vi "TLB Native Dynamic Events ver 0.07b.vi"() -> ()   [LabVIEW 2018]
uses:
  Labview Training Phase 2/Enum Controls/States for Action Engine.ctl
  Type def/TLB event states.ctl
  Type def/TLB MHL States.ctl
  <vilib>/Studica/Studica Toolkit/Background/I2C Channel.ctl
  <vilib>/Studica/Studica Toolkit/NavX/NavX.lvlib
  <vilib>/myRIO/Common/Instrument Driver Framework/myRIO v1.0/AI/typedefs/AI Channels Enum.ctl
  <vilib>/myRIO/Common/Instrument Driver Framework/myRIO v1.0/AI/typedefs/AI Channels List.ctl
  Type def/Type def.ctl
  Type def/Motor Control Cluster.ctl
  <vilib>/Studica/Studica Blackhawk/Blackhawk.lvlib
  <vilib>/userdefined/High Color/IMAQdx.ctl
  Underlying VI's/Webcam FGV Low level ver/State control.ctl
  <vilib>/Studica/Studica Toolkit/Background/Mxp Selection.ctl
  <vilib>/Studica/Studica Toolkit/Background/DIO Channel.ctl
  <vilib>/addons/control/pid/NI_PID_pid.lvlib
  <vilib>/addons/control/pid/pid.llb/PID (DBL).vi
  <vilib>/NI_Real-Time Target Support.lvlib
  <vilib>/ptbypt/NI_PtbyPt.lvlib
panel:
  out "Speed and distance cluster":T1
  out "Waveform Chart 2":dbl(graph)
  out "Load":errorcluster
  out "Waveform Chart":dbl(graph)
  in  "STOP":bool
  out "DIO 0":bool
  out "DIO 1":bool
  out "Limit Switch Array":bool[](array[boolean])
  out "error out":errorcluster
  out "L/R average":fxp<+,64,64>
  out "Right Ultrasonic":fxp<+,64,16>
  out "Left Ultrasonic":fxp<+,64,16>
  out "Object detection count":T2
  out "Camera error":errorcluster
  out "Right IR Sensor":dbl
  out "Left IR Sensor":dbl
  in  "Servo Angle":u8(slide) scale=0.0..180.0
  in  "On/Off":bool
  out "Blackhawk error":errorcluster
  out "element":T3
  out "Action Queue Items":i32
  out "State Logic Queue Items":i32
  out "Action Queues items":string[](array[string])=["Hardware reset", "Software reset", ""]
  out "State logic":T4=enum."Task 2"
  out "Action State":string
  in  "Tasks Selector":string(combo)="Drive straight"
  out "Yaw":dbl
  in  "NavX Zero Yaw":bool
  # "Camera Status Loop"
  # "TLB FRAMEWORK STATUS"
  # "Test Programme written by Calvin Loke    Dated: 28 Aug 2019\nTest Programme revised by Dr Alex See   Dated 30 Aug 2019\n\nProgramme version:   TLB Native Dynamic Events ver 0.04b.vi"
  # "Sequence of Actions"
  # "Continuous (Repeated)"
  # "Motor Control Loop"
  # "NAVX Control Loop"
  # "Sensor data"
  # "Blackhawk status"
  # "System Health Status Update"
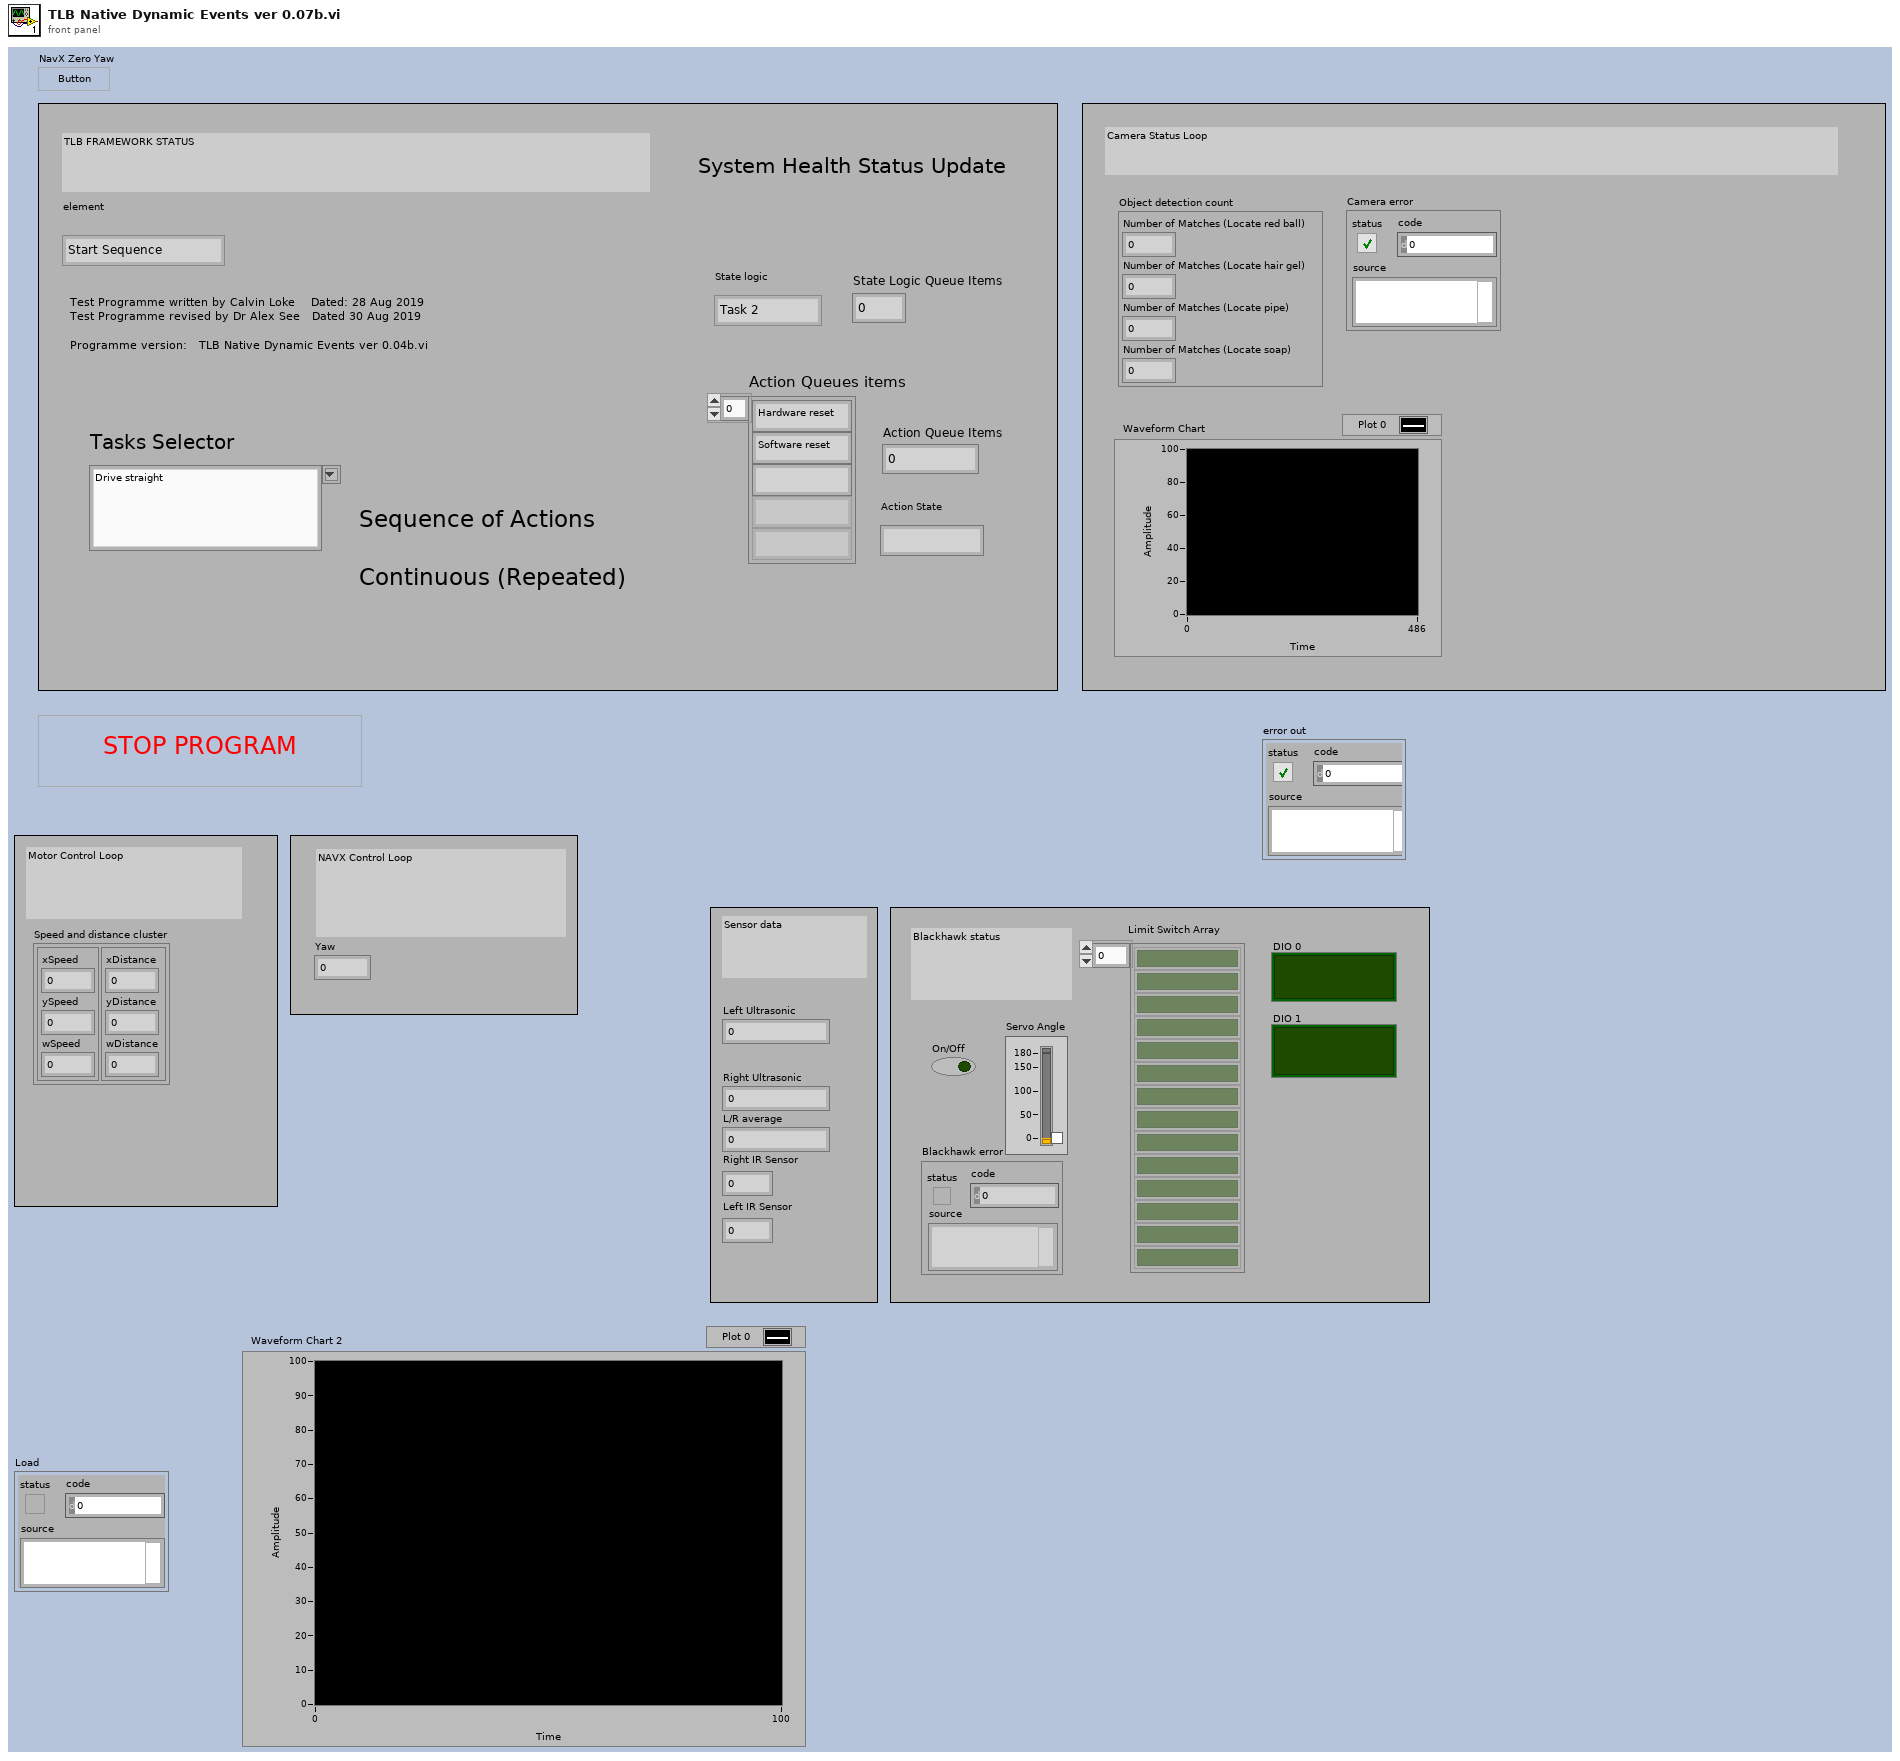
[diagram p1: front panel]
types:
  T1 = cluster{cluster{"xSpeed":dbl, "ySpeed":dbl, "wSpeed":dbl}, cluster{"xDistance":dbl, "yDistance":dbl, "wDistance":dbl}}
  T2 = cluster{"Number of Matches (Locate red ball)":i32, "Number of Matches (Locate hair gel)":i32, "Number of Matches (Locate pipe)":i32, "Number of Matches (Locate soap)":i32}
  T3 = typedef "TLB event states.ctl" = enum16{"Start Sequence", "Exit", "Start Task 1", "Start Task 2", "Start Task 3", "Start Task 4", "Camera vision", "Wall follow mode", "Idle", "Start Drive Straight"}
  T4 = typedef "TLB MHL States.ctl" = enum16{"None", "Startup", "Idle", "Processing", "Shutdown", "Reset", "Task 1", "Task 2", "Task 3", "Task 4", "Task 4a", "Task 4b", "Task 4c", "Task 4d", "Task 4e", "Task 4f", "Task 4g", "Task 4h", "Acquire image", "Wall follow mode", "Autodrive", "Autodrive a"}
  T5 = typedef "States for Action Engine.ctl" = enum16{"Initialize", "Write", "Read"}
  T6 = typedef "DIO Channel.ctl" = enum16{"Not Connected", "A/DIO1", "A/DIO2", "A/DIO3", "A/DIO4", "A/DIO5", "A/DIO6", "A/DIO7", "A/DIO13", "B/DIO1", "B/DIO2", "B/DIO3", "B/DIO4", "B/DIO5", "B/DIO6", "B/DIO7", "B/DIO13", "C/DIO0", "C/DIO1", "C/DIO2", "C/DIO3", "C/DIO4", "C/DIO5", "C/DIO6", "C/DIO7"}
  T7 = typedef "Motor Control Cluster.ctl" = cluster{"Vx":dbl, "Vy":dbl, "Vw":dbl}
  T8 = typedef "Type def.ctl" = cluster{"Front Ultrasonic Obstruct":bool, "Left Ultrasonic Obstruct":bool, "Right Ultrasonic Obstruct ":bool}
  T9 = typedef "I2C Channel.ctl" = enum16{"Not Connected", "A", "B"}
  T10 = typedef "TLB MHL States.ctl" = enum16{"None", "Startup", "Idle", "Processing", "Shutdown", "Reset", "Task 1", "Task 2", "Task 3", "Task 4", "Task 4a", "Task 4b", "Task 4c", "Task 4d", "Task 4e", "Task 4f", "Task 4g", "Task 4h", "Acquire image", "Wall follow mode", "Drive Straight"}
  T11 = cluster{"proportional gain (Kc)":dbl, "integral time (Ti, min)":dbl, "derivative time (Td, min)":dbl}
  T12 = typedef "State control.ctl" = enum16{"Initialise", "Start camera", "Continuous Acquisition ", "Stop camera", "Dispose all"}
  T13 = typedef "IMAQdx.ctl" = refnum<k21>
  T14 = typedef "Mxp Selection.ctl" = enum16{"MXP A", "MXP B"}
  T15 = cluster{"xTargetSpeed":dbl, "yTargetSpeed":dbl, "wTargetSpeed":dbl}
  T16 = typedef "IMAQ Image.ctl" = refnum<image>
  T17 = cluster{"xDistance":dbl, "yDistance":dbl, "wDistance":dbl}
  T18 = typedef "AI Channels List.ctl" = T19[]
  T19 = typedef "AI Channels Enum.ctl" = enum16{"Not Connected", "AudioIn/Left", "AudioIn/Right", "C/AI0", "C/AI1", "A/AI0", "A/AI1", "A/AI2", "A/AI3", "A/AI4", "A/AI5", "A/AI6", "A/AI7", "B/AI0", "B/AI1", "B/AI2", "B/AI3", "B/AI4", "B/AI5", "B/AI6", "B/AI7", "AI/AI0", "AI/AI1", "AI/AI2", "AI/AI3", "A/AI0 (DIFF)", "A/AI1 (DIFF)", "A/AI2 (DIFF)", "A/AI3 (DIFF)", "B/AI0 (DIFF)", "B/AI1 (DIFF)", "B/AI2 (DIFF)", "B/AI3 (DIFF)"}
  T20 = cluster{"I2C Ref Out":cluster{"I2C Channel":T9, "FPGA VI Reference Out":refnum<k20>}, "Connected":bool, "Slave Address (7-bit)":u8, "Registry":u8[]}
  T21 = cluster{"Yaw":dbl, "Roll":dbl, "Pitch":dbl, "Heading":dbl, "Fused Heading":dbl}
  T22 = cluster{"DIO Channel":T6, "FPGA VI Reference Out":refnum<k20>}
  T23 = cluster{"I2C Channel":T9, "FPGA VI Reference Out":refnum<k20>}
  T24 = typedef "NI_Real-Time Target Support.lvlib/RT CPU Load.ctl" = cluster{"Total (%)":dbl, "Time Critical (%)":dbl, "Timed Structures (%)":dbl, "High (%)":dbl, "Above Normal (%)":dbl, "Normal (%)":dbl, "Background (%)":dbl, "Idle (%)":dbl, "ISR (%)":dbl}
  T25 = cluster{"CPU loads[0]":T24, "CPU loads[1]":T24, "CPU loads[2]":T24, "CPU loads[3]":T24, "CPU loads[4]":T24, "CPU loads[5]":T24, "CPU loads[6]":T24, "CPU loads[7]":T24, "CPU loads[8]":T24}
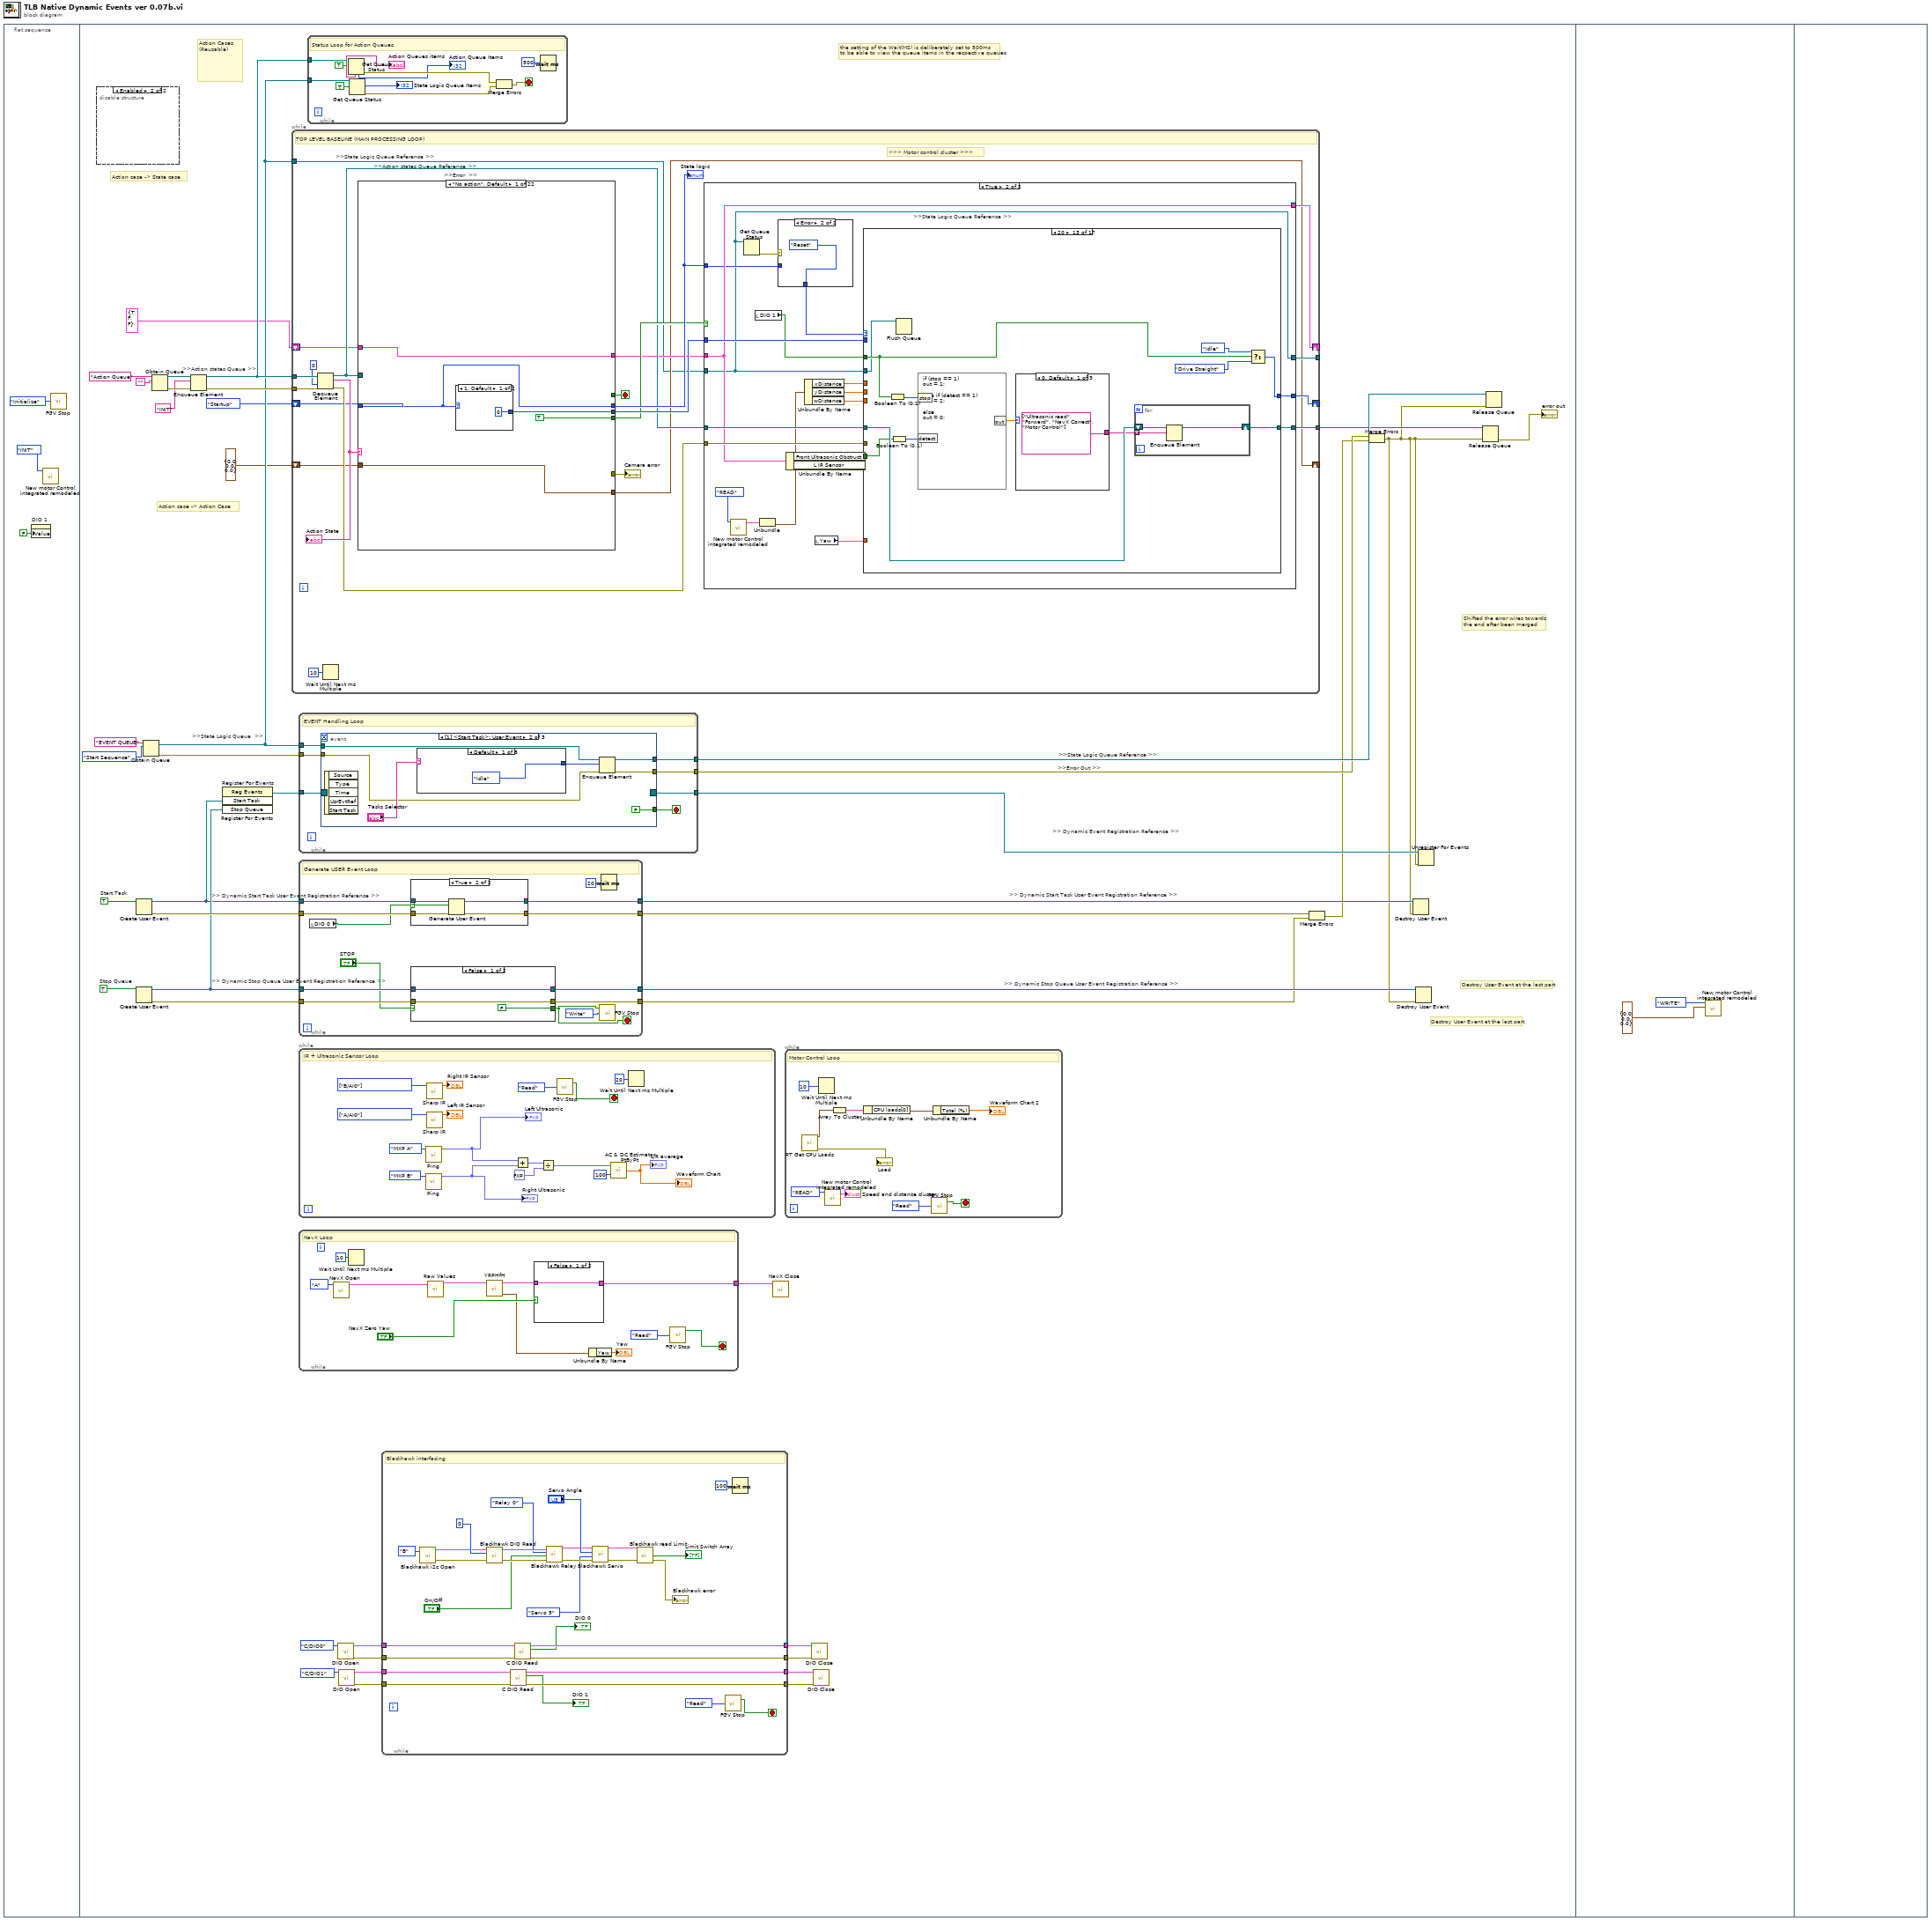
[diagram p0: block diagram]
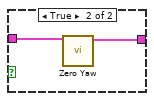
[diagram p2: hidden frame]
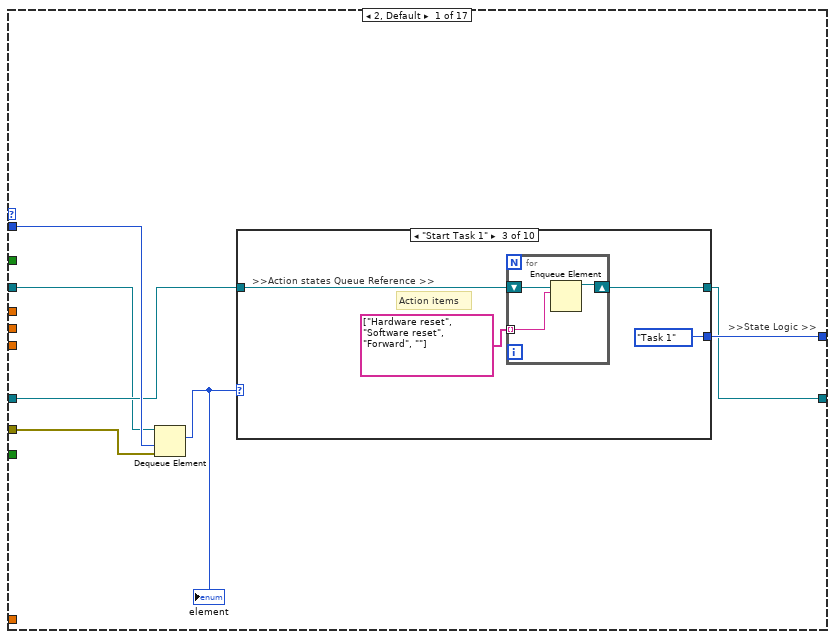
[diagram p5: hidden frame]
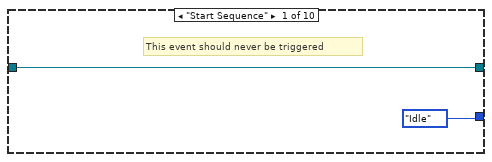
[diagram p6: hidden frame]
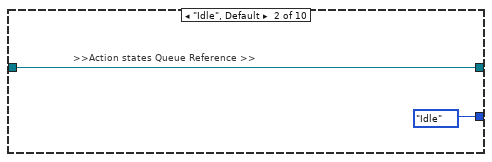
[diagram p7: hidden frame]
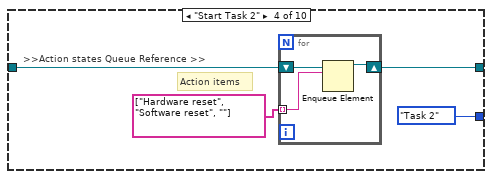
[diagram p8: hidden frame]
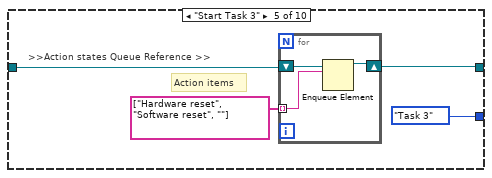
[diagram p9: hidden frame]
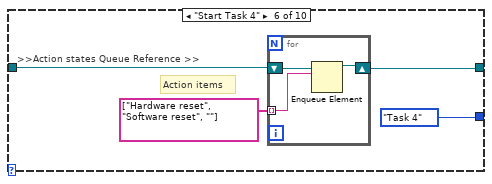
[diagram p10: hidden frame]
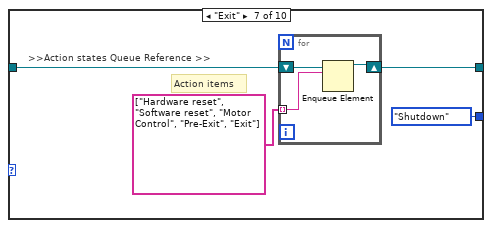
[diagram p11: hidden frame]
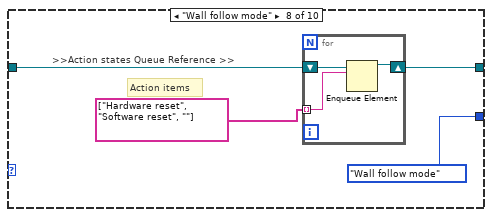
[diagram p12: hidden frame]
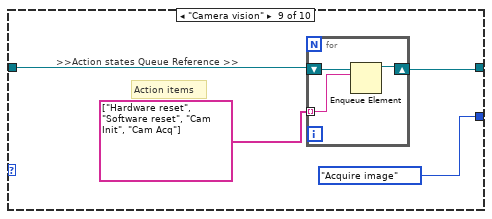
[diagram p13: hidden frame]
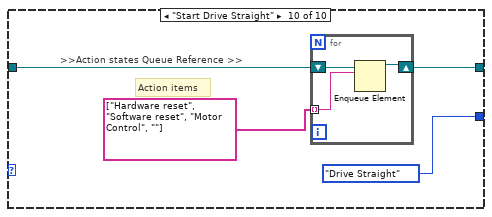
[diagram p14: hidden frame]
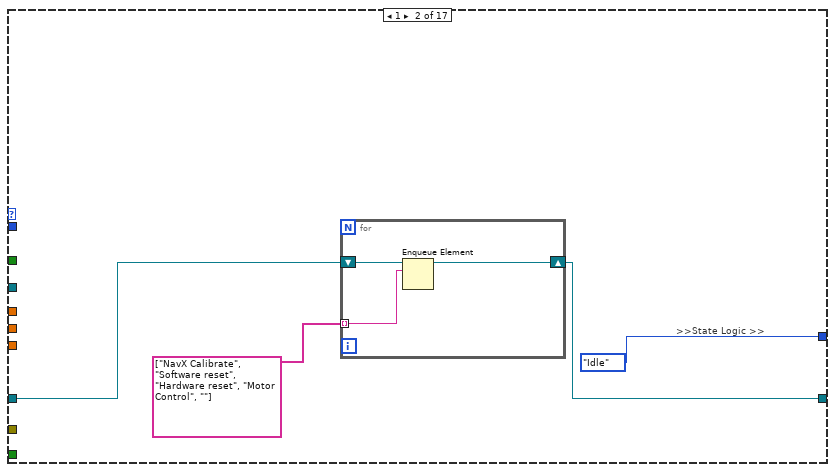
[diagram p15: hidden frame]
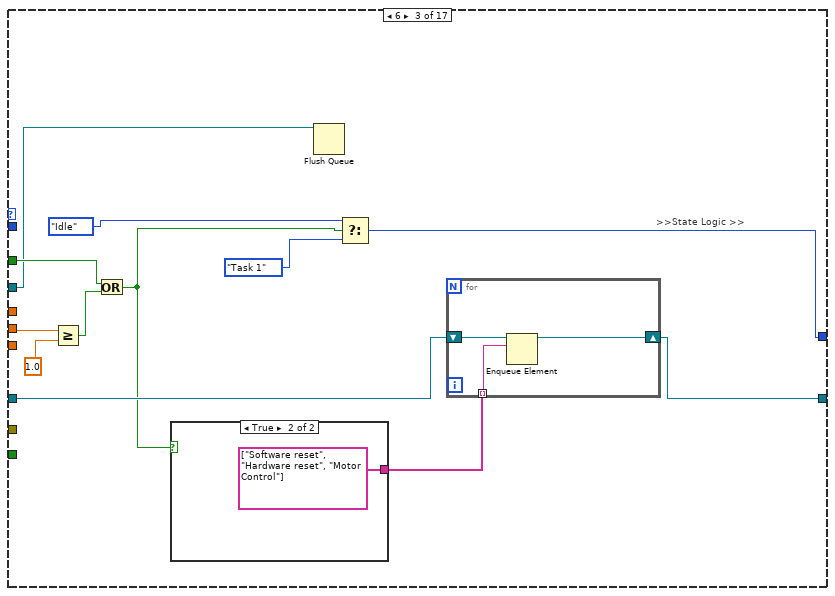
[diagram p16: hidden frame]
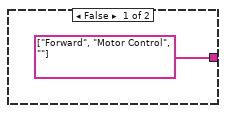
[diagram p17: hidden frame]
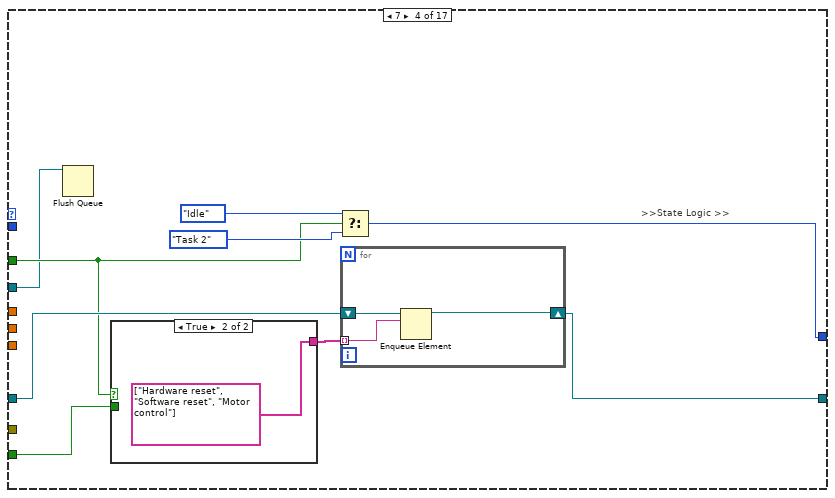
[diagram p18: hidden frame]
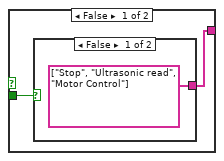
[diagram p19: hidden frame]
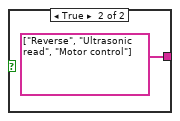
[diagram p20: hidden frame]
diagram:
  n1 = flat-sequence {
    frame #0 {
      n2 = property on="DIO 1" class="Bool (strict)"("Value"=FALSE ("DIO 1")) -> ()  [unwired: 2 in, 2 out]
      n3 = call "New motor Control integrated remodeled.vi"("States"=enum16{"RESET ENCODER", "WRITE", "READ", "INIT"}."INIT") -> ()  [unwired: 4 in, 2 out]
      n4 = call "FGV Stop.vi"("Init/Read/Write State"=States_for_Action_Engine."Initialize") -> ()  [unwired: 2 in, 2 out]
    }
    frame #1 {
      w46 = TRUE  # Stop Queue
      w45 = TRUE  # Start Task
      # "Action case -> Action Case"
      # "Action case -> State case"
      # "the setting of the Wait(MS) is deliberately set to 500ms\nto be able to view the queue items in the respective queues"
      # "Action Cases\n(Reusable)"
      # ">>Error Out >>"
      # ">> Dynamic Stop Queue User Event Registration Reference >>"
      # ">> Dynamic Start Task User Event Registration Reference >>"
      # ">> Dynamic Stop Queue User Event Registration Reference >>"
      # ">> Dynamic Start Task User Event Registration Reference >>"
      # ">> Dynamic Event Registration Reference >>"
      # ">>Action states Queue >>"
      # ">>State Logic Queue  >>"
      # ">>State Logic Queue Reference >>"
      # "Destroy User Event at the last part"
      # "Destroy User Event at the last part"
      # "Shifted the error wires towards\nthe end after been merged"
      n5 = disable-structure shown="Enabled" {
        frame Disabled {
          (unwired) variant
          (unwired) TRUE
          n6 = Variant To Data(type="") -> ()  [unwired: 2 in, 2 out]
        }
        frame Enabled {
        }
      }
      n7 = Create User Event(user event datatype=w45) -> (user event=w37:refnum<user-event>, error out=w42:errorcluster)  [unwired: 1 in]
      n8 = Create User Event(user event datatype=w46) -> (user event=w38:refnum<user-event>, error out=w41:errorcluster)  [unwired: 1 in]
      n9 = Obtain Queue(name (unnamed)="EVENT QUEUE", element data type=TLB_event_states."Start Sequence" ("Enum")) -> (queue out=w22:refnum<queue>, error out=w28:errorcluster)  [unwired: 3 in, 1 out]
      n10 = Obtain Queue(name (unnamed)="Action Queue", element data type="") -> (queue out=w31:refnum<queue>, error out=w27:errorcluster)  [unwired: 3 in, 1 out]
      n11 = Enqueue Element(queue=w31, element="INIT", error in (no error)=w27) -> (queue out=w23:refnum<queue>, error out=w26:errorcluster)  [unwired: 1 in, 1 out]
      n12 = register-events "Register For Events"(w37, w38) -> (reference out=w36:refnum<event-registration>)  [unwired: 2 in, 1 out]
      n13 = while {
        tunnel: w22 -> [w63]
        shift-right: [w76] -> _
        shift-left: TLB_MHL_States."Startup" ("Enum") -> [w70]
        tunnel: w23 -> [w81]
        tunnel: w26 -> [w79]
        tunnel: [w78] -> _
        tunnel: [w77] -> w17
        shift-right: [w67] -> _
        shift-left: T8 {"Front Ultrasonic Obstruct"=TRUE, "Left Ultrasonic Obstruct"=FALSE, "Right Ultrasonic Obstruct "=FALSE} -> [w69]
        shift-right: [w65] -> _
        shift-left: T7 {"Vx"=0.0, "Vy"=0.0, "Vw"=0.0} -> [w66]
        stop <- w61 stop-if-true
        # ">>> Motor control cluster >>>"
        # ">>Error  >>"
        # ">>Action states Queue Reference >>"
        # ">>State Logic Queue Reference >>"
        # "TOP LEVEL BASELINE (MAIN PROCESSING LOOP)"
        n14 = Dequeue Element(queue=w81, timeout in ms (-1)=0, error in (no error)=w79) -> (queue out=w71:refnum<queue>, element=w80:string, error out=w72:errorcluster)  [unwired: 1 out]
        "Action State" <- w80
        n15 = Wait Until Next ms Multiple(millisecond multiple=u32 10) -> ()  [unwired: 1 out]
        n16 = case shown="\"No action\", Default" w80 {
          tunnel: [w363 w375 w382 w390 w399 w407 w413 w423 w430 w436 w446 w456 TLB_MHL_States."Shutdown" ("Enum") w467 w477 w481 w496 w506 w519 w527 w541 w545] -> w82
          tunnel: [w367 0 0 0 0 0 0 0 0 0 0 0 0 0 0 0 0 0 0 0 0 0] -> w75
          tunnel: [TRUE FALSE FALSE FALSE FALSE FALSE FALSE FALSE FALSE FALSE FALSE FALSE FALSE FALSE FALSE FALSE FALSE FALSE FALSE FALSE FALSE FALSE] -> w74
          tunnel: w71 -> [_ _ _ _ _ _ _ _ _ _ _ _ _ _ _ _ _ _ _ _ _ _]
          tunnel: w70 -> [w363 w375 w382 w390 w399 w407 w413 w423 w430 w436 w446 w456 _ w467 w477 w481 w496 w506 w519 w527 w541 w545]
          tunnel: w69 -> [w365 w372 w379 w387 w395 w403 w411 w419 w427 w437 w443 w452 w459 w468 w476 w484 w497 w504 w520 w526 w537 w547]
          tunnel: [w365 w372 w379 w387 w395 w403 w411 w419 w427 w437 w442 w452 w459 w468 w473 w483 w497 w504 w520 w526 w537 w547] -> w68
          tunnel: w66 -> [w364 w371 w377 w385 w393 w402 w409 w418 w425 w433 w440 w451 w458 w464 w470 w478 w492 w507 w518 w530 w538 w546]
          tunnel: [w364 w371 w378 w386 w394 w401 w410 w417 w426 w433 w440 w449 w458 w464 w470 w478 w493 w508 w518 w530 w538 w546] -> w65
          tunnel: [_ _ _ _ _ _ _ _ _ _ _ _ _ _ _ _ _ _ w509 w522 w531 _] -> w64
          tunnel: [_ _ _ _ _ _ _ _ _ _ _ _ TRUE _ _ _ _ _ _ _ _ _] -> w61
          frame "No action", Default {
            n17 = case shown="1, Default" w363 {
              tunnel: [0 100] -> w367
              frame 1, Default {
              }
              frame 2 {
              }
            }
          }
          frame "Init" {
            # ">>State Logic  >>"
            n18 = local write "Servo Angle"(u8 90 ("Servo Angle")) -> ()
          }
          frame "Forward" {
            n19 = local write "NavX Zero Yaw"(FALSE ("NavX Zero Yaw")) -> ()
            n20 = Bundle By Name(cluster=w377, "Vy"=0.6) -> (w378:T7)
          }
          frame "Reverse" {
            n21 = local write "NavX Zero Yaw"(FALSE ("NavX Zero Yaw")) -> ()
            n22 = Bundle By Name(cluster=w385, "Vy"=-0.6) -> (w386:T7)
          }
          frame "Right" {
            n23 = local write "NavX Zero Yaw"(FALSE ("NavX Zero Yaw")) -> ()
            n24 = Bundle By Name(cluster=w393, "Vx"=0.6) -> (w394:T7)
          }
          frame "Left" {
            n25 = Bundle By Name(cluster=w402, "Vx"=-0.6) -> (w401:T7)
            n26 = local write "NavX Zero Yaw"(FALSE ("NavX Zero Yaw")) -> ()
          }
          frame "Rotate CW" {
            n27 = local write "NavX Zero Yaw"(FALSE ("NavX Zero Yaw")) -> ()
            n28 = Bundle By Name(cluster=w409, "Vw"=-0.3) -> (w410:T7)
          }
          frame "Rotate ACW" {
            n29 = local write "NavX Zero Yaw"(FALSE ("NavX Zero Yaw")) -> ()
            n30 = Bundle By Name(cluster=w418, "Vw"=0.15) -> (w417:T7)
          }
          frame "Stop" {
            w424 = 0.0
            n31 = local write "NavX Zero Yaw"(FALSE ("NavX Zero Yaw")) -> ()
            n32 = Bundle By Name(cluster=w425, "Vx"=w424, "Vy"=w424, "Vw"=w424) -> (w426:T7)
          }
          frame "Motor control" {
            n33 = call "New motor Control integrated remodeled.vi"("States"=enum16{"RESET ENCODER", "WRITE", "READ", "INIT"}."WRITE", "Target Speed"=w433) -> ()  [unwired: 3 in, 2 out]
          }
          frame "Software reset" {
            w441 = FALSE ("NavX Zero Yaw")
            n34 = Wait (ms)(milliseconds to wait=u32 20) -> ()  [unwired: 1 out]
            n35 = local write "NavX Zero Yaw"(w441) -> ()
            n36 = Bundle By Name(cluster=w443, "Front Ultrasonic Obstruct"=w441, "L IR Sensor"=0.0) -> (w442:T8)
          }
          frame "Hardware reset" {
            w450 = 0.0
            n37 = Wait (ms)(milliseconds to wait=u32 20) -> ()  [unwired: 1 out]
            n38 = local write "NavX Zero Yaw"(TRUE ("NavX Zero Yaw")) -> ()
            n39 = call "New motor Control integrated remodeled.vi"("States"=enum16{"RESET ENCODER", "WRITE", "READ", "INIT"}."RESET ENCODER") -> ()  [unwired: 4 in, 2 out]
            n40 = Bundle By Name(cluster=w451, "Vx"=w450, "Vy"=w450, "Vw"=w450) -> (w449:T7)
          }
          frame "Exit" {
          }
          frame "Pre-Exit" {
            n41 = call "New motor Control integrated remodeled.vi"("States"=enum16{"RESET ENCODER", "WRITE", "READ", "INIT"}."INIT") -> ()  [unwired: 4 in, 2 out]
          }
          frame "Ultrasonic read" {
            # "Object detection"
            n42 = local read "L/R average"() -> (w469:fxp<+,64,64>)
            n43 = Less Or Equal?(x=w469, y=35.0) -> (x <= y?=w471:bool)
            n44 = Bundle By Name(cluster=w476, "Front Ultrasonic Obstruct"=w471) -> (w473:T8)
          }
          frame "IR Sensor Read" {
            n45 = local read "Left IR Sensor"() -> (w482:dbl)
            n46 = Bundle By Name(cluster=w484, "L IR Sensor"=w482) -> (w483:T8)
          }
          frame "Calculate" {
            n47 = Unbundle By Name(w497) -> ("L IR Sensor"=w489:dbl)
            n48 = call-poly <vilib>:"PID.vi"("output range"=cluster{"output high":dbl, "output low":dbl} {"output high"=0.3, "output low"=-0.3}, "PID gains"=T11 {"proportional gain (Kc)"=0.01, "integral time (Ti, min)"=0.0, "derivative time (Td, min)"=0.0}, "process variable"=w489, "setpoint"=20.0) -> ("output"=w486:dbl)  [unwired: 6 in, 1 out]
            n49 = Negate(x=w486) -> (-x=w485:dbl)
            n50 = Bundle By Name(cluster=w492, "Vy"=0.2, "Vw"=w485) -> (w493:T7)
          }
          frame "NavX Correct" {
            n51 = local read "Yaw"() -> (w501:dbl)
            n52 = call-poly <vilib>:"PID.vi"("output range"=cluster{"output high":dbl, "output low":dbl} {"output high"=0.1, "output low"=-0.1}, "PID gains"=T11 {"proportional gain (Kc)"=0.1, "integral time (Ti, min)"=0.001, "derivative time (Td, min)"=0.0}, "process variable"=w501, "setpoint"=0.0 ("y")) -> ("output"=w498:dbl)  [unwired: 6 in, 1 out]
            n53 = Bundle By Name(cluster=w507, "Vw"=w498) -> (w508:T7)
          }
          frame "Cam Init" {
            n54 = call "Low-Level Grab.vi"("States"=State_control."Initialise", "Session In"=T13 "cam1") -> ("error out"=w510:errorcluster, "Session Out"=w511:T13)  [unwired: 7 in, 1 out]
            n55 = call "Low-Level Grab.vi"("error in (no error)"=w510, "States"=State_control."Start camera", "Session In"=w511) -> ("error out"=w509:errorcluster)  [unwired: 6 in, 2 out]
            n56 = local write "Servo Angle"(u8 170 ("Servo Angle")) -> ()
          }
          frame "Cam Acq" {
            n57 = call "Low-Level Grab.vi"("States"=State_control."Continuous Acquisition ") -> ("error out"=w523:errorcluster, "Image Out"=w524:T16)  [unwired: 8 in, 1 out]
            n58 = call "All object detection ver2.vi"("Image In"=w524, "error in"=w523) -> ("Object detection count"=→"Object detection count":T2, "error out"=w522:errorcluster)  [unwired: 1 out]
          }
          frame "Cam Exit" {
            n59 = call "Low-Level Grab.vi"("States"=State_control."Stop camera") -> ("error out"=w532:errorcluster, "Session Out"=w534:T13)  [unwired: 8 in, 1 out]
            n60 = call "Low-Level Grab.vi"("error in (no error)"=w532, "States"=State_control."Dispose all", "Session In"=w534) -> ("error out"=w531:errorcluster)  [unwired: 6 in, 2 out]
            n61 = local write "Servo Angle"(u8 90 ("Servo Angle")) -> ()
          }
          frame "NavX Calibrate" {
            n62 = Wait (ms)(milliseconds to wait=u32 20000) -> ()  [unwired: 1 out]
          }
        }
        "State logic" <- w82
        "Camera error" <- w64
        n63 = case shown="True" w74 {
          tunnel: w82 -> [w85 w90]
          tunnel: w63 -> [w86 w89]
          tunnel: w71 -> [w84 w105]
          tunnel: [w86 w89] -> w78
          tunnel: [w84 w104] -> w77
          tunnel: [w85 w103] -> w76
          tunnel: w72 -> [_ w102]
          tunnel: w75 -> [_ w101]
          tunnel: w68 -> [w83 w95]
          tunnel: [w83 w95] -> w67
          frame False {
          }
          frame True {
            # ">>State Logic Queue Reference >>"
            n64 = call "New motor Control integrated remodeled.vi"("States"=enum16{"RESET ENCODER", "WRITE", "READ", "INIT"}."READ") -> ("Speed and distance cluster"=w94:T1)  [unwired: 4 in, 1 out]
            n65 = Get Queue Status(queue=w89) -> (error out=w88:errorcluster)  [unwired: 2 in, 7 out]
            n66 = local read "DIO 1"() -> (w87:bool)
            n67 = Unbundle(w94) -> (w93:T17)  [unwired: 1 out]
            n68 = case shown="Error" w88 {
              tunnel: [w106 TLB_MHL_States."Reset" ("Enum")] -> w91
              tunnel: w90 -> [w106 _]
              frame No Error {
              }
              frame Error {
              }
            }
            n69 = Unbundle By Name(w95) -> ("Front Ultrasonic Obstruct"=w96:bool)  [unwired: 1 out]
            n70 = Unbundle By Name(w93) -> ("xDistance"=w98:dbl, "yDistance"=w100:dbl, "wDistance"=w99:dbl)
            n71 = local read "Yaw"() -> (w97:dbl)
            n72 = case shown="20" w91 {
              tunnel: w89 -> [w108 _ w182 w199 _ _ _ _ _ w286 _ w308 w321 w339 _ _ _]
              tunnel: w105 -> [w110 w176 w189 w203 w225 w234 w248 w263 w276 w292 w302 w311 w328 w343 w352 w355 w361]
              tunnel: [w109 w175 w188 w204 w224 w235 w247 w262 w275 w291 w301 w312 w329 w342 w352 w354 w361] -> w104
              tunnel: [w113 TLB_MHL_States."Idle" ("Enum") w191 w205 w221 w238 w250 w261 w277 w290 TLB_MHL_States."Shutdown" ("Enum") w314 w330 w341 TLB_MHL_States."Reset" ("Enum") TLB_MHL_States."Shutdown" ("Enum") TLB_MHL_States."Reset" ("Enum")] -> w103
              tunnel: w102 -> [w111 _ _ _ _ _ _ _ _ _ _ _ _ _ _ _ _]
              tunnel: w101 -> [w112 _ _ _ _ _ _ _ _ _ _ _ _ _ _ _ _]
              tunnel: w87 -> [_ _ w186 w202 w219 _ _ _ _ w289 _ w309 w326 w340 _ _ _]
              tunnel: w100 -> [_ _ w183 _ _ _ _ w258 _ _ _ _ _ _ _ _ _]
              tunnel: w99 -> [_ _ _ _ w216 _ _ _ _ _ _ _ _ _ _ _ _]
              tunnel: w98 -> [_ _ _ _ _ _ w244 _ w272 _ _ _ _ _ _ _ _]
              tunnel: w97 -> [_ _ _ _ _ _ _ _ _ _ _ _ _ _ _ _ _]
              tunnel: w96 -> [_ _ _ w200 _ w232 _ _ _ w288 _ _ w323 _ _ _ _]
              frame 2, Default {
                # ">>State Logic >>"
                n73 = Dequeue Element(queue=w108, timeout in ms (-1)=w112, error in (no error)=w111) -> (element=w114:T3)  [unwired: 3 out]
                "element" <- w114
                n74 = case shown="\"Start Task 1\"" w114 {
                  tunnel: [TLB_MHL_States."Idle" ("Enum") TLB_MHL_States."Idle" ("Enum") TLB_MHL_States."Task 1" ("Enum") TLB_MHL_States."Task 2" ("Enum") TLB_MHL_States."Task 3" ("Enum") TLB_MHL_States."Task 4" ("Enum") TLB_MHL_States."Shutdown" ("Enum") TLB_MHL_States."Wall follow mode" ("Enum") TLB_MHL_States."Acquire image" ("Enum") TLB_MHL_States."Drive Straight" ("Enum")] -> w113
                  tunnel: [w116 w117 w121 w126 w135 w141 w147 w154 w162 w169] -> w109
                  tunnel: w110 -> [w116 w117 w119 w127 w136 w142 w148 w155 w163 w170]
                  frame "Start Sequence" {
                    # "This event should never be triggered"
                  }
                  frame "Idle", Default {
                    # ">>Action states Queue Reference >>"
                  }
                  frame "Start Task 1" {
                    # ">>Action states Queue Reference >>"
                    # "Action items"
                    n75 = for {
                      shift-right: [w125] -> w121
                      shift-left: w119 -> [w124]
                      tunnel: string[] ["Hardware reset", "Software reset", "Forward", ""] -> [w123] mode=indexing
                      n76 = Enqueue Element(queue=w124, element=w123) -> (queue out=w125:refnum<queue>)  [unwired: 2 in, 2 out]
                    }
                  }
                  frame "Start Task 2" {
                    # ">>Action states Queue Reference >>"
                    # "Action items"
                    n77 = for {
                      shift-right: [w132] -> w126
                      shift-left: w127 -> [w131]
                      tunnel: string[] ["Hardware reset", "Software reset", ""] -> [w130] mode=indexing
                      n78 = Enqueue Element(queue=w131, element=w130) -> (queue out=w132:refnum<queue>)  [unwired: 2 in, 2 out]
                    }
                  }
                  frame "Start Task 3" {
                    # ">>Action states Queue Reference >>"
                    # "Action items"
                    n79 = for {
                      shift-right: [w139] -> w135
                      shift-left: w136 -> [w138]
                      tunnel: string[] ["Hardware reset", "Software reset", ""] -> [w137] mode=indexing
                      n80 = Enqueue Element(queue=w138, element=w137) -> (queue out=w139:refnum<queue>)  [unwired: 2 in, 2 out]
                    }
                  }
                  frame "Start Task 4" {
                    # ">>Action states Queue Reference >>"
                    # "Action items"
                    n81 = for {
                      shift-right: [w146] -> w141
                      shift-left: w142 -> [w145]
                      tunnel: string[] ["Hardware reset", "Software reset", ""] -> [w144] mode=indexing
                      n82 = Enqueue Element(queue=w145, element=w144) -> (queue out=w146:refnum<queue>)  [unwired: 2 in, 2 out]
                    }
                  }
                  frame "Exit" {
                    # ">>Action states Queue Reference >>"
                    # "Action items"
                    n83 = for {
                      shift-right: [w153] -> w147
                      shift-left: w148 -> [w152]
                      tunnel: string[] ["Hardware reset", "Software reset", "Motor Control", "Pre-Exit", "Exit"] -> [w151] mode=indexing
                      n84 = Enqueue Element(queue=w152, element=w151) -> (queue out=w153:refnum<queue>)  [unwired: 2 in, 2 out]
                    }
                  }
                  frame "Wall follow mode" {
                    # ">>Action states Queue Reference >>"
                    # "Action items"
                    n85 = for {
                      shift-right: [w160] -> w154
                      shift-left: w155 -> [w159]
                      tunnel: string[] ["Hardware reset", "Software reset", ""] -> [w158] mode=indexing
                      n86 = Enqueue Element(queue=w159, element=w158) -> (queue out=w160:refnum<queue>)  [unwired: 2 in, 2 out]
                    }
                  }
                  frame "Camera vision" {
                    # ">>Action states Queue Reference >>"
                    # "Action items"
                    n87 = for {
                      shift-right: [w167] -> w162
                      shift-left: w163 -> [w166]
                      tunnel: string[] ["Hardware reset", "Software reset", "Cam Init", "Cam Acq"] -> [w165] mode=indexing
                      n88 = Enqueue Element(queue=w166, element=w165) -> (queue out=w167:refnum<queue>)  [unwired: 2 in, 2 out]
                    }
                  }
                  frame "Start Drive Straight" {
                    # ">>Action states Queue Reference >>"
                    # "Action items"
                    n89 = for {
                      shift-right: [w174] -> w169
                      shift-left: w170 -> [w173]
                      tunnel: string[] ["Hardware reset", "Software reset", "Motor Control", ""] -> [w172] mode=indexing
                      n90 = Enqueue Element(queue=w173, element=w172) -> (queue out=w174:refnum<queue>)  [unwired: 2 in, 2 out]
                    }
                  }
                }
              }
              frame 1 {
                # ">>State Logic >>"
                n91 = for {
                  shift-right: [w180] -> w175
                  shift-left: w176 -> [w181]
                  tunnel: string[] ["NavX Calibrate", "Software reset", "Hardware reset", "Motor Control", ""] -> [w179] mode=indexing
                  n92 = Enqueue Element(queue=w181, element=w179) -> (queue out=w180:refnum<queue>)  [unwired: 2 in, 2 out]
                }
              }
              frame 6 {
                # ">>State Logic >>"
                n93 = Greater Or Equal?(x=w183, y=1.0) -> (x >= y?=w184:bool)
                n94 = Or(x=w186, y=w184) -> (x .or. y?=w187:bool)
                n95 = case shown="True" w187 {
                  tunnel: [string[] ["Forward", "Motor Control", ""] string[] ["Software reset", "Hardware reset", "Motor Control"]] -> w190
                  frame False {
                  }
                  frame True {
                  }
                }
                n96 = Flush Queue(queue=w182) -> ()  [unwired: 1 in, 3 out]
                n97 = Select(t=TLB_MHL_States."Idle" ("Enum"), s=w187, f=TLB_MHL_States."Task 1" ("Enum")) -> (s? t:f=w191:T4)
                n98 = for {
                  shift-right: [w197] -> w188
                  shift-left: w189 -> [w198]
                  tunnel: w190 -> [w196] mode=indexing
                  n99 = Enqueue Element(queue=w198, element=w196) -> (queue out=w197:refnum<queue>)  [unwired: 2 in, 2 out]
                }
              }
              frame 7 {
                # ">>State Logic >>"
                n100 = Flush Queue(queue=w199) -> ()  [unwired: 1 in, 3 out]
                n101 = case shown="True" w202 {
                  tunnel: [w209 string[] ["Hardware reset", "Software reset", "Motor control"]] -> w201
                  tunnel: w200 -> [w208 _]
                  frame False {
                    n102 = case shown="False" w208 {
                      tunnel: [string[] ["Stop", "Ultrasonic read", "Motor Control"] string[] ["Reverse", "Ultrasonic read", "Motor control"]] -> w209
                      frame False {
                      }
                      frame True {
                      }
                    }
                  }
                  frame True {
                  }
                }
                n103 = Select(t=TLB_MHL_States."Idle" ("Enum"), s=w202, f=TLB_MHL_States."Task 2" ("Enum")) -> (s? t:f=w205:T4)
                n104 = for {
                  shift-right: [w214] -> w204
                  shift-left: w203 -> [w215]
                  tunnel: w201 -> [w213] mode=indexing
                  n105 = Enqueue Element(queue=w215, element=w213) -> (queue out=w214:refnum<queue>)  [unwired: 2 in, 2 out]
                }
              }
              frame 8 {
                n106 = Less Or Equal?(x=w216, y=-1.2) -> (x <= y?=w217:bool)
                n107 = Or(x=w217, y=w219) -> (x .or. y?=w220:bool)
                n108 = case shown="True" w220 {
                  tunnel: [string[] ["Rotate CW", "Motor Control"] string[] ["Software reset", "Hardware reset", "Motor Control"]] -> w226
                  frame False {
                  }
                  frame True {
                  }
                }
                n109 = for {
                  shift-right: [w228] -> w224
                  shift-left: w225 -> [w229]
                  tunnel: w226 -> [w227] mode=indexing
                  n110 = Enqueue Element(queue=w229, element=w227) -> (queue out=w228:refnum<queue>)  [unwired: 2 in, 2 out]
                }
                n111 = Select(t=TLB_MHL_States."Idle" ("Enum"), s=w220, f=TLB_MHL_States."Task 3" ("Enum")) -> (s? t:f=w221:T4)
              }
              frame 9 {
                n112 = case shown="True" w232 {
                  tunnel: [string[] ["Forward", "Ultrasonic read", "Motor Control"] string[] ["Stop", "Hardware reset", "Software reset", "Motor Control"]] -> w233
                  frame False {
                  }
                  frame True {
                  }
                }
                n113 = for {
                  shift-right: [w242] -> w235
                  shift-left: w234 -> [w243]
                  tunnel: w233 -> [w241] mode=indexing
                  n114 = Enqueue Element(queue=w243, element=w241) -> (queue out=w242:refnum<queue>)  [unwired: 2 in, 2 out]
                }
                n115 = Select(t=TLB_MHL_States."Task 4a" ("Enum"), s=w232, f=TLB_MHL_States."Task 4" ("Enum")) -> (s? t:f=w238:T4)
              }
              frame 10 {
                n116 = Greater Or Equal?(x=w244, y=0.5) -> (x >= y?=w246:bool)
                n117 = case shown="True" w246 {
                  tunnel: [string[] ["Right", "Motor Control"] string[] ["Stop", "Hardware reset", "Software reset", "Motor Control"]] -> w249
                  frame False {
                  }
                  frame True {
                  }
                }
                n118 = for {
                  shift-right: [w256] -> w247
                  shift-left: w248 -> [w257]
                  tunnel: w249 -> [w255] mode=indexing
                  n119 = Enqueue Element(queue=w257, element=w255) -> (queue out=w256:refnum<queue>)  [unwired: 2 in, 2 out]
                }
                n120 = Select(t=TLB_MHL_States."Task 4b" ("Enum"), s=w246, f=TLB_MHL_States."Task 4a" ("Enum")) -> (s? t:f=w250:T4)
              }
              frame 11 {
                n121 = Greater Or Equal?(x=w258, y=0.75) -> (x >= y?=w259:bool)
                n122 = case shown="False" w259 {
                  tunnel: [string[] ["Forward", "Motor control"] string[] ["Stop", "Hardware reset", "Software reset"]] -> w264
                  frame False {
                  }
                  frame True {
                  }
                }
                n123 = for {
                  shift-right: [w270] -> w262
                  shift-left: w263 -> [w271]
                  tunnel: w264 -> [w269] mode=indexing
                  n124 = Enqueue Element(queue=w271, element=w269) -> (queue out=w270:refnum<queue>)  [unwired: 2 in, 2 out]
                }
                n125 = Select(t=TLB_MHL_States."Task 4c" ("Enum"), s=w259, f=TLB_MHL_States."Task 4b" ("Enum")) -> (s? t:f=w261:T4)
              }
              frame 12 {
                n126 = Less Or Equal?(x=w272, y=-0.65) -> (x <= y?=w273:bool)
                n127 = case shown="False" w273 {
                  tunnel: [string[] ["Left", "Motor Control"] string[] ["Stop", "Hardware reset", "Software reset", "Motor Control"]] -> w278
                  frame False {
                  }
                  frame True {
                  }
                }
                n128 = for {
                  shift-right: [w284] -> w275
                  shift-left: w276 -> [w285]
                  tunnel: w278 -> [w283] mode=indexing
                  n129 = Enqueue Element(queue=w285, element=w283) -> (queue out=w284:refnum<queue>)  [unwired: 2 in, 2 out]
                }
                n130 = Select(t=TLB_MHL_States."Task 4d" ("Enum"), s=w273, f=TLB_MHL_States."Task 4c" ("Enum")) -> (s? t:f=w277:T4)
              }
              frame 13 {
                n131 = Flush Queue(queue=w286) -> ()  [unwired: 1 in, 3 out]
                n132 = Or(x=w289, y=w288) -> (x .or. y?=w287:bool)
                n133 = case shown="True" w287 {
                  tunnel: [string[] ["Forward", "Ultrasonic Read", "Motor Control"] string[] ["Stop", "Hardware reset", "Software reset", "Motor Control"]] -> w293
                  frame False {
                  }
                  frame True {
                  }
                }
                n134 = for {
                  shift-right: [w299] -> w291
                  shift-left: w292 -> [w300]
                  tunnel: w293 -> [w298] mode=indexing
                  n135 = Enqueue Element(queue=w300, element=w298) -> (queue out=w299:refnum<queue>)  [unwired: 2 in, 2 out]
                }
                n136 = Select(t=TLB_MHL_States."Idle" ("Enum"), s=w287, f=TLB_MHL_States."Task 4d" ("Enum")) -> (s? t:f=w290:T4)
              }
              frame 5 {
                n137 = for {
                  shift-right: [w306] -> w301
                  shift-left: w302 -> [w307]
                  tunnel: string[] ["Software reset", "Hardware reset", "Motor Control"] -> [w305] mode=indexing
                  n138 = Enqueue Element(queue=w307, element=w305) -> (queue out=w306:refnum<queue>)  [unwired: 2 in, 2 out]
                }
              }
              frame 19 {
                n139 = Flush Queue(queue=w308) -> ()  [unwired: 1 in, 3 out]
                n140 = case shown="False" w309 {
                  tunnel: [string[] ["IR Sensor Read", "Calculate", "Forward", "Motor Control"] string[] ["Hardware reset", "Software reset", "Motor Control"]] -> w310
                  frame False {
                  }
                  frame True {
                  }
                }
                n141 = for {
                  shift-right: [w319] -> w312
                  shift-left: w311 -> [w320]
                  tunnel: w310 -> [w318] mode=indexing
                  n142 = Enqueue Element(queue=w320, element=w318) -> (queue out=w319:refnum<queue>)  [unwired: 2 in, 2 out]
                }
                n143 = Select(t=TLB_MHL_States."Idle" ("Enum"), s=w309, f=TLB_MHL_States."Wall follow mode" ("Enum")) -> (s? t:f=w314:T4)
              }
              frame 20 {
                n144 = Boolean To (0,1)(Boolean=w326) -> (0, 1=w325:i16)
                n145 = Boolean To (0,1)(Boolean=w323) -> (0, 1=w324:i16)
                n146 = Flush Queue(queue=w321) -> ()  [unwired: 1 in, 3 out]
                n147 = formula code="if (stop == 1)\nout = 1;\n\nelse if (detect == 1)\nout = 2;\n\nelse \nout = 0;"("stop"=w325, "detect"=w324) -> ("out"=w327:dbl)
                n148 = case shown="0, Default" w327 {
                  tunnel: [string[] ["Ultrasonic read", "Forward", "NavX Correct", "Motor Control"] string[] ["Hardware reset", "Software reset", "Motor Control"] string[] ["Stop", "Motor Control", "Ultrasonic read"]] -> w322
                  frame 0, Default {
                  }
                  frame 1 {
                  }
                  frame 2 {
                  }
                }
                n149 = for {
                  shift-right: [w337] -> w329
                  shift-left: w328 -> [w338]
                  tunnel: w322 -> [w336] mode=indexing
                  n150 = Enqueue Element(queue=w338, element=w336) -> (queue out=w337:refnum<queue>)  [unwired: 2 in, 2 out]
                }
                n151 = Select(t=TLB_MHL_States."Idle" ("Enum"), s=w326, f=TLB_MHL_States."Drive Straight" ("Enum")) -> (s? t:f=w330:u16)
              }
              frame 18 {
                n152 = Flush Queue(queue=w339) -> ()  [unwired: 1 in, 3 out]
                n153 = case shown="True" w340 {
                  tunnel: [string[] ["Cam Acq"] string[] ["Hardware reset", "Software reset", "Cam Exit", ""]] -> w344
                  frame False {
                  }
                  frame True {
                  }
                }
                n154 = for {
                  shift-right: [w350] -> w342
                  shift-left: w343 -> [w351]
                  tunnel: w344 -> [w349] mode=indexing
                  n155 = Enqueue Element(queue=w351, element=w349) -> (queue out=w350:refnum<queue>)  [unwired: 2 in, 2 out]
                }
                n156 = Select(t=TLB_MHL_States."Idle" ("Enum"), s=w340, f=TLB_MHL_States."Acquire image" ("Enum")) -> (s? t:f=w341:T4)
              }
              frame 3 {
              }
              frame 4 {
                # ">>State Logic >>"
                n157 = for {
                  shift-right: [w359] -> w354
                  shift-left: w355 -> [w360]
                  tunnel: string[] ["Software reset", "Hardware reset", "Motor Control", "Cam Exit", "Pre-Exit", "Exit"] -> [w358] mode=indexing
                  n158 = Enqueue Element(queue=w360, element=w358) -> (queue out=w359:refnum<queue>)  [unwired: 2 in, 2 out]
                }
              }
              frame 0 {
              }
            }
          }
        }
      }
      n159 = while {
        tunnel: w36 -> [w582]
        tunnel: [w581] -> w35
        tunnel: w22 -> [w579]
        tunnel: [w578] -> w34
        tunnel: w28 -> [w577]
        tunnel: [w576] -> w25
        stop <- w580 stop-if-true
        # "EVENT Handling Loop"
        n160 = event shown="[1] <Start Task>: User Event" {
          selector: w582 -> [_ _ _]
          dyn-events: [_ _ _] -> w581
          timeout: _ -> [_ _ _]
          tunnel: [FALSE FALSE w609] -> w580
          tunnel: w579 -> [w587 w594 w607]
          tunnel: [w586 w593 w608] -> w578
          tunnel: w577 -> [w584 w590 w605]
          tunnel: [w583 w589 w604] -> w576
          event Timeout {
            n161 = event-data() -> ()  [unwired: 1 in, 3 out]
            n162 = Enqueue Element(queue=w587, element=TLB_event_states."Idle" ("Enum"), error in (no error)=w584) -> (queue out=w586:refnum<queue>, error out=w583:errorcluster)  [unwired: 1 in, 1 out]
          }
          event User Event {
            n163 = event-data() -> ()  [unwired: 1 in, 5 out]
            n164 = case shown="Default" "Tasks Selector" {
              tunnel: [TLB_event_states."Idle" ("Enum") TLB_event_states."Start Task 1" ("Enum") TLB_event_states."Start Task 2" ("Enum") TLB_event_states."Start Task 3" ("Enum") TLB_event_states."Start Task 4" ("Enum") TLB_event_states."Wall follow mode" ("Enum") TLB_event_states."Camera vision" ("Enum") TLB_event_states."Start Drive Straight" ("Enum")] -> w591
              frame Default {
              }
              frame "Task 1" {
              }
              frame "Task 2" {
              }
              frame "Task 3" {
              }
              frame "Task 4" {
              }
              frame "Wall following" {
              }
              frame "RT Camera tracking" {
              }
              frame "Drive straight" {
              }
            }
            n165 = Enqueue Element(queue=w594, element=w591, error in (no error)=w590) -> (queue out=w593:refnum<queue>, error out=w589:errorcluster)  [unwired: 1 in, 1 out]
          }
          event User Event {
            n166 = event-data() -> ("Stop Queue"=w609:bool)  [unwired: 1 in, 4 out]
            n167 = Enqueue Element At Opposite End(queue=w607, element=TLB_event_states."Exit" ("Enum"), error in (no error)=w605) -> (queue out=w608:refnum<queue>, error out=w604:errorcluster)  [unwired: 1 in, 1 out]
          }
        }
      }
      n168 = while {
        tunnel: w37 -> [w621]
        tunnel: w38 -> [w620]
        tunnel: [w619] -> w44
        tunnel: [w618] -> w43
        tunnel: w42 -> [w617]
        tunnel: [w616] -> w40
        tunnel: w41 -> [w615]
        tunnel: [w614] -> w39
        stop <- w612 stop-if-true
        # "Generate USER Event Loop"
        n169 = local read "DIO 0"() -> (w611:bool)
        n170 = case shown="True" w611 {
          selector: w611 -> [_ w633]
          tunnel: w621 -> [w632 w637]
          tunnel: [w632 w636] -> w618
          tunnel: w617 -> [w631 w635]
          tunnel: [w631 w634] -> w616
          frame False {
          }
          frame True {
            n171 = Generate User Event(user event=w637, event data cluster=w633, error in=w635) -> (user event out=w636:refnum<user-event>, error out=w634:errorcluster)  [unwired: 1 in]
          }
        }
        n172 = case shown="False" "STOP" {
          selector: "STOP" -> [_ w626]
          tunnel: w620 -> [w625 w630]
          tunnel: [w625 w629] -> w619
          tunnel: w615 -> [w624 w628]
          tunnel: [w624 w627] -> w614
          tunnel: [FALSE w626] -> w612
          frame False {
          }
          frame True {
            n173 = Generate User Event(user event=w630, event data cluster=w626, error in=w628) -> (user event out=w629:refnum<user-event>, error out=w627:errorcluster)  [unwired: 1 in]
          }
        }
        n174 = call "FGV Stop.vi"("Init/Read/Write State"=States_for_Action_Engine."Write", "Input Node"=w612) -> ()  [unwired: 1 in, 2 out]
        n175 = Wait (ms)(milliseconds to wait=u32 20) -> ()  [unwired: 1 out]
      }
      n176 = while {
        stop <- w558 stop-if-true
        w563 = T18 [enum."A/AI0"] items=["Not Connected", "AudioIn/Left", "AudioIn/Right", "C/AI0", "C/AI1", "A/AI0", "A/AI1", "A/AI2", "A/AI3", "A/AI4", "A/AI5", "A/AI6", "A/AI7", "B/AI0", "B/AI1", "B/AI2", "B/AI3", "B/AI4", "B/AI5", "B/AI6", "B/AI7", "AI/AI0", "AI/AI1", "AI/AI2", "AI/AI3", "A/AI0 (DIFF)", "A/AI1 (DIFF)", "A/AI2 (DIFF)", "A/AI3 (DIFF)", "B/AI0 (DIFF)", "B/AI1 (DIFF)", "B/AI2 (DIFF)", "B/AI3 (DIFF)"] ("AI Channel")
        w564 = T18 [enum."B/AI0"] items=["Not Connected", "AudioIn/Left", "AudioIn/Right", "C/AI0", "C/AI1", "A/AI0", "A/AI1", "A/AI2", "A/AI3", "A/AI4", "A/AI5", "A/AI6", "A/AI7", "B/AI0", "B/AI1", "B/AI2", "B/AI3", "B/AI4", "B/AI5", "B/AI6", "B/AI7", "AI/AI0", "AI/AI1", "AI/AI2", "AI/AI3", "A/AI0 (DIFF)", "A/AI1 (DIFF)", "A/AI2 (DIFF)", "A/AI3 (DIFF)", "B/AI0 (DIFF)", "B/AI1 (DIFF)", "B/AI2 (DIFF)", "B/AI3 (DIFF)"] ("AI Channel")
        # "IR + Ultrasonic Sensor Loop"
        n177 = call <vilib>:"Ping.vi"("Mxp Side"=Mxp_Selection."MXP B") -> ("CM"=w552:fxp<+,64,16>)  [unwired: 8 in, 2 out]
        "Right Ultrasonic" <- w552
        n178 = call <vilib>:"Ping.vi"("Mxp Side"=Mxp_Selection."MXP A") -> ("CM"=w553:fxp<+,64,16>)  [unwired: 8 in, 2 out]
        "Left Ultrasonic" <- w553
        n179 = call <vilib>:"Sharp IR.vi"("AI Channel"=w564) -> ("Sharp IR Distance"=→"Right IR Sensor":dbl)  [unwired: 8 in, 2 out]
        n180 = call <vilib>:"Sharp IR.vi"("AI Channel"=w563) -> ("Sharp IR Distance"=→"Left IR Sensor":dbl)  [unwired: 8 in, 2 out]
        n181 = Add(x=w553, y=w552) -> (x+y=w555:fxp<+,64,17>)
        n182 = Divide(x=w555, y=fxp<+,64,17> 2.0) -> (x/y=w551:fxp<+,64,64>)
        n183 = call "FGV Stop.vi"("Init/Read/Write State"=States_for_Action_Engine."Read") -> ("Output node"=w558:bool)  [unwired: 2 in, 1 out]
        n184 = call <vilib>:"AC & DC Estimator PtByPt.vi"("signal"=w551, "sample length"=100) -> ("DC estimate (V)"=→"L/R average" →"Waveform Chart":dbl)  [unwired: 1 in, 2 out]
        n185 = Wait Until Next ms Multiple(millisecond multiple=u32 20) -> ()  [unwired: 1 out]
      }
      n186 = while {
        tunnel: [w49] -> w14
        stop <- w56 stop-if-true
        # "NavX Loop"
        n187 = call <vilib>:"NavX Open.vi"("I2C Channel"=I2C_Channel."A") -> ("NavX Info"=w47:T20)  [unwired: 9 in, 1 out]
        n188 = Wait Until Next ms Multiple(millisecond multiple=u32 10) -> ()  [unwired: 1 out]
        n189 = call <vilib>:"Raw Values.vi"("NavX Info In"=w47) -> ("NavX Info Out"=w51:T20)  [unwired: 8 in, 1 out]
        n190 = call <vilib>:"YRPHfH.vi"("NavX Info In"=w51) -> ("YRPHfH"=w53:T21, "NavX Info Out"=w50:T20)  [unwired: 3 in]
        n191 = case shown="False" "NavX Zero Yaw" {
          tunnel: [w58 w60] -> w49
          tunnel: w50 -> [w58 w59]
          frame False {
          }
          frame True {
            n192 = call <vilib>:"Zero Yaw.vi"("NavX Info In"=w59) -> ("NavX Info Out"=w60:T20)  [unwired: 10 in]
          }
        }
        n193 = Unbundle By Name(w53) -> ("Yaw"=→"Yaw":dbl)
        n194 = call "FGV Stop.vi"("Init/Read/Write State"=States_for_Action_Engine."Read") -> ("Output node"=w56:bool)  [unwired: 2 in, 1 out]
      }
      n195 = while {
        tunnel: w23 -> [w573]
        tunnel: w22 -> [w570]
        stop <- w567 stop-if-true
        # "Status Loop for Action Queues"
        n196 = Get Queue Status(queue=w573, return elements? (F)=TRUE) -> (error out=w569:errorcluster, # elements in queue=→"Action Queue Items":i32, elements=→"Action Queues items":string[])  [unwired: 1 in, 5 out]
        n197 = Get Queue Status(queue=w570, return elements? (F)=TRUE) -> (# pending remove=→"State Logic Queue Items":i32, error out=w568:errorcluster)  [unwired: 1 in, 6 out]
        n198 = Merge Errors(w569, w568) -> (w567:errorcluster)
        n199 = Wait (ms)(milliseconds to wait=u32 500) -> ()  [unwired: 1 out]
      }
      n200 = call <vilib>:"DIO Open.vi"("DIO Channel"=DIO_Channel."C/DIO0") -> ("error out"=w7:errorcluster, "DIO Info Out"=w13:T22)  [unwired: 9 in]
      n201 = call <vilib>:"DIO Open.vi"("DIO Channel"=DIO_Channel."C/DIO1") -> ("error out"=w5:errorcluster, "DIO Info Out"=w9:T22)  [unwired: 9 in]
      n202 = while {
        tunnel: w13 -> [w660]
        tunnel: [w659] -> w12
        tunnel: w9 -> [w658]
        tunnel: [w657] -> w8
        tunnel: w7 -> [w656]
        tunnel: [w655] -> w6
        tunnel: w5 -> [w654]
        tunnel: [w653] -> w4
        stop <- w674 stop-if-true
        # "Blackhawk interfacing"
        n203 = call <vilib>:"Blackhawk i2c Open.vi"("I2C Channel"=I2C_Channel."B") -> ("I2C Ref Out"=w649:T23, "error out"=w648:errorcluster)  [unwired: 2 in]
        n204 = call <vilib>:"Blackhawk DIO Read.vi"("I2C Ref In"=w649, "PIN"=u8 0, "error in (no error)"=w648) -> ("I2C Ref Out"=w672:T23, "error out"=w673:errorcluster)  [unwired: 3 in, 1 out]
        n205 = call <vilib>:"C DIO Read.vi"("error in (no error)"=w654, "DIO Info In in"=w658) -> ("error out"=w653:errorcluster, "IN"=→"DIO 1":bool, "DIO Info In out"=w657:T22)  [unwired: 7 in]
        n206 = call <vilib>:"C DIO Read.vi"("error in (no error)"=w656, "DIO Info In in"=w660) -> ("error out"=w655:errorcluster, "IN"=→"DIO 0":bool, "DIO Info In out"=w659:T22)  [unwired: 7 in]
        n207 = call <vilib>:"Blackhawk Relay.vi"("error in (no error)"=w673, "On/Off"="On/Off", "Relay"=enum8{"Relay 0", "Relay 1", "Relay 2"}."Relay 0", "I2C Ref In"=w672) -> ("error out"=w669:errorcluster, "I2C Ref Out"=w666:T23)  [unwired: 6 in]
        n208 = call <vilib>:"Blackhawk Servo.vi"("error in (no error)"=w669, "Servo Select"=enum16{"Servo 5", "Servo 6"}."Servo 5", "Servo Angle"="Servo Angle", "I2C Ref In"=w666) -> ("error out"=w664:errorcluster, "I2C Ref Out"=w663:T23)  [unwired: 6 in]
        n209 = call <vilib>:"Blackhawk read Limit.vi"("error in (no error)"=w664, "I2C Ref In"=w663) -> ("error out"=→"Blackhawk error":errorcluster, "Limit Switch Array"=→"Limit Switch Array":bool[])  [unwired: 1 in, 1 out]
        n210 = call "FGV Stop.vi"("Init/Read/Write State"=States_for_Action_Engine."Read") -> ("Output node"=w674:bool)  [unwired: 2 in, 1 out]
        n211 = Wait (ms)(milliseconds to wait=u32 100) -> ()  [unwired: 1 out]
      }
      n212 = call <vilib>:"NavX Close.vi"("NavX Info In"=w14) -> ()  [unwired: 10 in, 1 out]
      n213 = while {
        stop <- w645 stop-if-true
        # "Motor Control Loop"
        n214 = call <vilib>:"RT Get CPU Loads.vi"() -> ("error out"=→"Load":errorcluster, "CPU loads"=w642:T24[])  [unwired: 10 in]
        n215 = Wait Until Next ms Multiple(millisecond multiple=u32 10) -> ()  [unwired: 1 out]
        n216 = call "New motor Control integrated remodeled.vi"("States"=enum16{"RESET ENCODER", "WRITE", "READ", "INIT"}."READ") -> ("Speed and distance cluster"=→"Speed and distance cluster":T1)  [unwired: 4 in, 1 out]
        n217 = Array To Cluster(array=w642) -> (cluster=w641:T25)
        n218 = Unbundle By Name(w641) -> ("CPU loads[0]"=w640:T24)
        n219 = call "FGV Stop.vi"("Init/Read/Write State"=States_for_Action_Engine."Read") -> ("Output node"=w645:bool)  [unwired: 2 in, 1 out]
        n220 = Unbundle By Name(w640) -> ("Total (%)"=→"Waveform Chart 2":dbl)
      }
      n221 = call <vilib>:"DIO Close.vi"("error in (no error)"=w6, "DIO Info In"=w12) -> ()  [unwired: 9 in, 1 out]
      n222 = call <vilib>:"DIO Close.vi"("error in (no error)"=w4, "DIO Info In"=w8) -> ()  [unwired: 9 in, 1 out]
      n223 = Merge Errors "Merge Errors"(w40, w39) -> (w21:errorcluster)
      n224 = Merge Errors(w25, w21) -> (w15:errorcluster)
      n225 = Destroy User Event(user event=w43, error in=w15) -> ()  [unwired: 1 out]
      n226 = Destroy User Event(user event=w44, error in=w15) -> ()  [unwired: 1 out]
      n227 = Unregister For Events(event registration refnum=w35, error in=w15) -> ()  [unwired: 1 out]
      n228 = Release Queue(queue=w17, error in (no error)=w15) -> (error out=→"error out":errorcluster)  [unwired: 1 in, 2 out]
      n229 = Release Queue(queue=w34, error in (no error)=w15) -> ()  [unwired: 1 in, 3 out]
    }
    frame #2 {
      n230 = call "New motor Control integrated remodeled.vi"("States"=enum16{"RESET ENCODER", "WRITE", "READ", "INIT"}."WRITE", "Target Speed"=T15 {"xTargetSpeed"=0.0, "yTargetSpeed"=0.0, "wTargetSpeed"=0.0}) -> ()  [unwired: 3 in, 2 out]
    }
    frame #3 {
    }
  }
